vi "test xilinx divider.vi"() -> ()   [LabVIEW 2015]
uses:
  <vilib>/Platform/TimedLoop/XDataNode/timing_clust.ctl
  <vilib>/Platform/TimedLoop/XDataNode/nitl_modes.ctl
  <vilib>/Platform/TimedLoop/XDataNode/wakeup.ctl
  <vilib>/rvi/IPIntegrationNode/IPINode_Typedef/niFpgaIPINodeSupportedFamilies.ctl
  <vilib>/rvi/Emulation/niFpgaSctlEmulationGetInTimedLoop.vi
  <vilib>/rvi/Emulation/niFpgaEmulationReportErrorSimple.vi
  <vilib>/rvi/Emulation/niFpgaGetClockAttributes.vi
  <vilib>/rvi/Emulation/niFpgaCriticalErrorInLSC.vi
  <vilib>/rvi/IPIntegrationNode/IPINode_Utilities/niFpgaIPINodeSimCore.vi
  <vilib>/Platform/TimedLoop/XDataNode/XDataNode.xnode
  <vilib>/rvi/XilinxIP/XIPIN_XNode/niFpgaXIPIN.xnode
  C:/Bitbucket/si5/scanimage-secondary/SI5 LabVIEW FPGA/coregen/DivideSGLCH0 1/DivideSGLCH0_1_A744216CC47F4488B8B32F92EAF8224F.dll
  <vilib>/rvi/IPIntegrationNode/IPINode_Xnode/niFpgaIPINode.xnode
  <vilib>/Platform/TimedLoop/XDataNode/XDNodeRunTimeDep.lvlib
panel:
  in  "Input (I32) 2":i32
  in  "Input (I32)":i32
  out "result 2":sgl
  in  "clk":bool
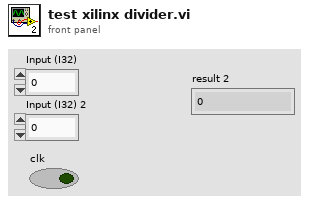
[diagram p1: front panel]
types:
  T1 = typedef "XDNodeRunTimeDep.lvlib/timing_clust.ctl" = cluster{"Expected End [f-1]":u64, "Actual End [f-1]":u64, "Finished Late? [f-1]":bool, "Expected End [i-1]":u64, "Actual End [i-1]":u64, "Finished Late? [i-1]":bool, "Expected Start [i]":u64, "Actual Start [i]":u64, "Expected Start [f]":u64, "Actual Start [f]":u64, "Source Name":string, "Structure Name":string, "Period":i64, "Deadline":i64, "Offset":i64, "Start":i64, "Priority":i32, "Timeout":i32, "Mode":T2, "Wakeup Reason":T3, "Error":errorcluster, "Source Type":string, "Secondary Source Type":string, "Global End Time":u64, "Global Start Time":u64, "Frame Duration":u64, "Iteration Duration":u64, "Assigned CPU":i32, "I/O Scan Engine Mode":u32}
  T2 = typedef "XDNodeRunTimeDep.lvlib/nitl_modes.ctl" = enum32{"No Change", "Process missed periods, maintain original phase", "Discard missed periods, maintain original phase", "Process missed periods, ignore original phase", "Discard missed periods, ignore original phase"}
  T3 = typedef "XDNodeRunTimeDep.lvlib/wakeup.ctl" = enum32{"Normal", "Aborted", "Asynchronous wakeup", "Timing source error", "Timed loop error", "Timeout"}
  T4 = typedef "niFpgaIPINodeSupportedFamilies.ctl" = cluster{"unlimited?":bool, "supported targets":string[]}
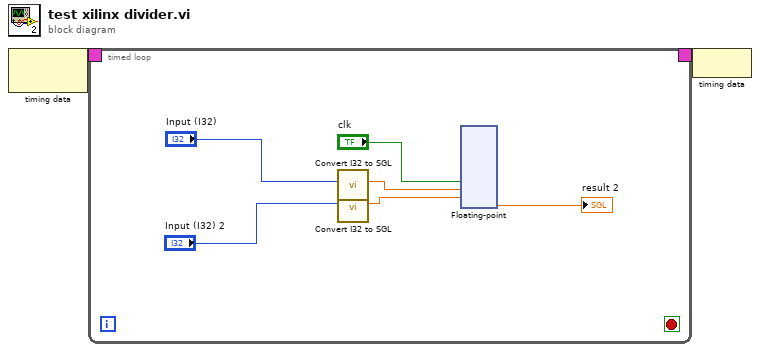
[diagram p0: block diagram]
diagram:
  n1 = node-c288() -> (w2:T1)  [unwired: 1 in]
  n2 = timed-loop {
    timing: w2 -> [_]
    timing-out: [_] -> w1
    stop <- _ stop-if-true
    n3 = call "Convert I32 to SGL.vi"("Input (I32)"="Input (I32)") -> ("Output (SGL)"=w8:sgl)  [unwired: 9 in, 1 out]
    n4 = call "Convert I32 to SGL.vi"("Input (I32)"="Input (I32) 2") -> ("Output (SGL)"=w7:sgl)  [unwired: 9 in, 1 out]
    n5 = xnode ("Floating-point")("clk"="clk", "a"=w8, "b"=w7) -> ("result"=→"result 2":sgl)
  }
  n6 = node-c288(w1) -> ()
